vi "ziModStatus.vi"(7 "Error In":errorcluster, 10 "ModHandle IN":T1 {"ModHandle" format="0x%08x"; "Conn" format="0x%08x"}) -> (0 "Error Out":errorcluster, 1 "Finished?":bool, 2 "Progress (unity)":dbl, 3 "ModHandle Out":T1 {"ModHandle" format="0x%08x"; "Conn" format="0x%08x"})   [LabVIEW 2015, in "Zurich Instruments LabOne.lvlib"]
doc: "This vi gives the status of the Module run and returns a finished flag when the module has finished."
uses:
  Zurich Instruments LabOne.lvlib
  Zurich Instruments/LabOne/API/LabVIEW/Zurich Instruments LabOne/Private/ziLV64.framework
  ziTypeModHandle.ctl
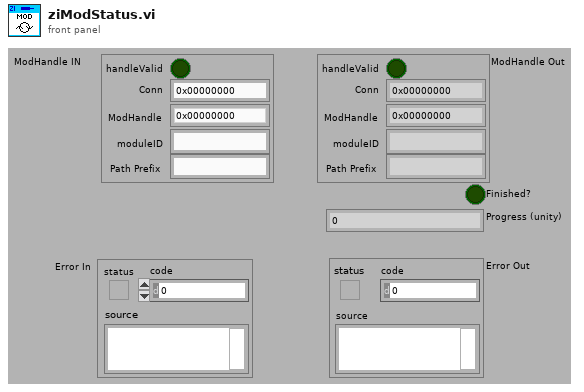
[diagram p1: front panel]
types:
  T1 = typedef "Zurich Instruments LabOne.lvlib/ziTypeModHandle.ctl" = cluster{"handleValid":bool, "Conn":u64, "ModHandle":u64, "moduleID":string, "Path Prefix":string}
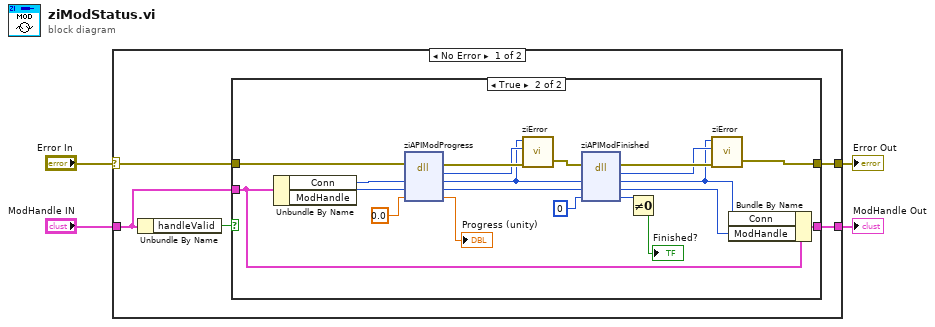
[diagram p0: block diagram]
diagram:
  n1 = case shown="No Error" "Error In" {
    selector: "Error In" -> [w7 w33]
    tunnel: "ModHandle IN" -> [w6 w32]
    tunnel: [w9 w32] -> w1
    tunnel: [w8 w33] -> w4
    frame No Error {
      n2 = Unbundle By Name(w6) -> ("handleValid"=w5:bool)
      n3 = case shown="True" w5 {
        tunnel: w6 -> [w11 w31]
        tunnel: [w11 w30] -> w9
        tunnel: w7 -> [w10 w25]
        tunnel: [w10 w28] -> w8
        frame False {
        }
        frame True {
          n4 = Unbundle By Name(w31) -> ("Conn"=w26:u64, "ModHandle"=w27:u64)
          n5 = dll-call lib="Users/arkady/Desktop/ado/github/resonant_ultrasound_arxiv/maglab ultrasound -- arkady --arxiv/Zurich Instruments/LabOne/API/LabVIEW/Zurich Instruments LabOne/Private/ziLV*.*" fn="ziAPIModProgress"(error in=w25, "conn"=w26, "ModHandle"=w27, "Finished"=0.0) -> (error out=w21:errorcluster, "return type"=w19:u32, "conn"=w13:u64, "ModHandle"=w24:u64, "Finished"=→"Progress (unity)":dbl)  [unwired: 2 in, 1 out]
          n6 = call "ziError.vi"("Conn"=w13, "ziErrorCode"=w19, "Error In"=w21) -> ("Error Out"=w20:errorcluster)  [unwired: 2 in, 1 out]
          n7 = dll-call lib="Users/arkady/Desktop/ado/github/resonant_ultrasound_arxiv/maglab ultrasound -- arkady --arxiv/Zurich Instruments/LabOne/API/LabVIEW/Zurich Instruments LabOne/Private/ziLV*.*" fn="ziAPIModFinished"(error in=w20, "conn"=w13, "ModHandle"=w24, "Finished"=i64 0) -> (error out=w18:errorcluster, "return type"=w17:u32, "conn"=w12:u64, "ModHandle"=w29:u64, "Finished"=w22:i64)  [unwired: 2 in, 1 out]
          n8 = Not Equal To 0?(x=w22) -> (x != 0?=→"Finished?":bool)
          n9 = call "ziError.vi"("Conn"=w12, "ziErrorCode"=w17, "Error In"=w18) -> ("Error Out"=w28:errorcluster)  [unwired: 2 in, 1 out]
          n10 = Bundle By Name(cluster=w31, "Conn"=w12, "ModHandle"=w29) -> (w30:T1)
        }
      }
    }
    frame Error {
    }
  }
  "Error Out" <- w4
  "ModHandle Out" <- w1
